vi "Servo.vi"(8 "Angle (deg)":dbl=45.0, 9 "Servo Pin":u16(ring)=1 items=["X1"=1], 11 "Data In":T1) -> (3 "Data Out":T1={"Port"="", "All Code"="Hi"})   [LabVIEW 2016]
uses:
  uPythonX/PythonData.ctl
  uPythonX/uPythonX.xctl
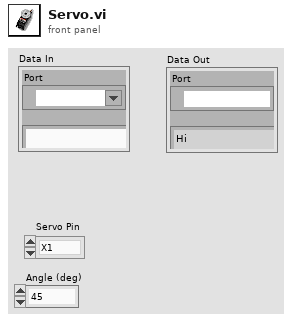
[diagram p1: front panel]
types:
  T1 = typedef "uPythonX.xctl/PythonData.ctl" = cluster{"Port":refnum<visa-resource-name>, "All Code":string}
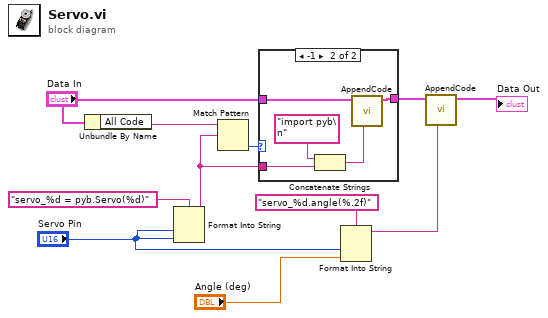
[diagram p0: block diagram]
diagram:
  n1 = Unbundle By Name("Data In") -> ("All Code"=w9:string)
  n2 = Format Into String(format string="servo_%d = pyb.Servo(%d)", "Servo Pin", "Servo Pin") -> (resulting string=w6:string)  [unwired: 2 in, 1 out]
  n3 = Match Pattern(string=w9, regular expression=w6) -> (offset past match=w8:i32)  [unwired: 1 in, 3 out]
  n4 = case shown="-1" w8 {
    tunnel: "Data In" -> [w12 w17]
    tunnel: w6 -> [_ w14]
    tunnel: [w12 w16] -> w5
    frame Default {
    }
    frame -1 {
      n5 = Concatenate Strings("import pyb\n" ("format string"), w14) -> (w13:string)
      n6 = call "AppendCode.vi"("New Code"=w13, "Data In"=w17) -> ("Data Out"=w16:T1)  [unwired: 9 in]
    }
  }
  n7 = Format Into String(format string="servo_%d.angle(%.2f)", "Servo Pin", "Angle (deg)") -> (resulting string=w3:string)  [unwired: 2 in, 1 out]
  n8 = call "AppendCode.vi"("New Code"=w3, "Data In"=w5) -> ("Data Out"=→"Data Out":T1)  [unwired: 9 in]
